vi "ToDatagram.vi"(8 "error in (no error)":errorcluster, 10 "messageID":u16, 11 "PingResponseMqttMsg in":refnum<class "PingResponseMqttMsg.lvclass">) -> (0 "error out":errorcluster, 2 "Datagram":u8[](array[numeric]), 3 "PingResponseMqttMsg out":refnum<class "PingResponseMqttMsg.lvclass">)   [LabVIEW 2020, in "PingResponseMqttMsg.lvclass"]
uses:
  PingResponseMqttMsg.lvclass
  mqttTypedef/MessageType.ctl
  mqttTypedef/QosLevel.ctl
  BaseMqttMsg.lvclass
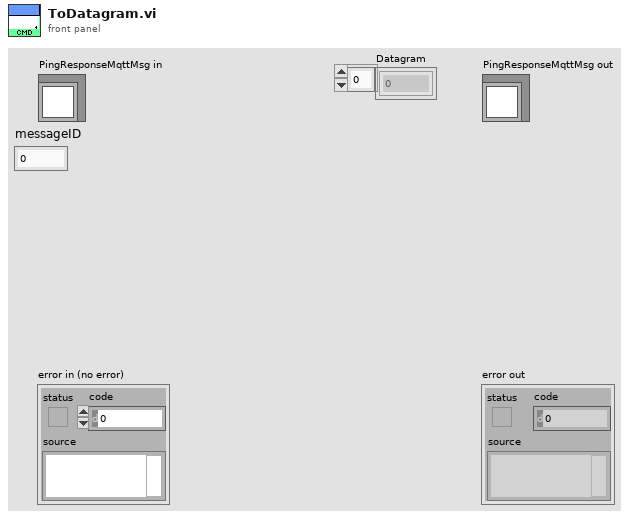
[diagram p1: front panel]
types:
  T1 = typedef "BaseMqttMsg.lvclass/QosLevel.ctl" = enum8{"At most once", "At least once", "Exactly once", "Reserved"}
  T2 = typedef "BaseMqttMsg.lvclass/MessageType.ctl" = enum32{"Reserved", "CONNECT", "CONNACK", "PUBLISH", "PUBACK", "PUBREC", "PUBREL", "PUBCOMP", "SUBSCRIBE", "SUBACK", "UNSUBSCRIBE", "UNSUBACK", "PINGREQ", "PINGRESP", "DISCONNECT", "Reserved2"}
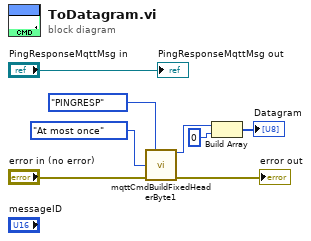
[diagram p0: block diagram]
diagram:
  n1 = call "mqttCmdBuildFixedHeaderByte1.vi"("MessageType"=MessageType."PINGRESP", "QoS (At most once)"=QosLevel."At most once", "error in (no error)"="error in (no error)") -> ("byte1"=w6:u8, "error out"=→"error out":errorcluster)  [unwired: 11 in]
  n2 = Build Array(w6, u8 0 ("byte1")) -> (→"Datagram":u8[])
  "PingResponseMqttMsg out" <- "PingResponseMqttMsg in"
